vi "UHR-Fleezers Control (fpga) - 10.0.vi"() -> ()   [LabVIEW 2009]
doc: "UHR-Fleezers Instrument Control Code (fpga)"
uses:
  <vilib>/Platform/TimedLoop/XDataNode/XDataNode.xnode
  <vilib>/Platform/TimedLoop/XDataNode/loadlvalarms.vi
  <vilib>/Platform/TimedLoop/XDataNode/timing_clust.ctl
  <vilib>/Platform/TimedLoop/XDataNode/nitl_modes.ctl
  <vilib>/Platform/TimedLoop/XDataNode/wakeup.ctl
  <vilib>/eio/EIONode/EIONode.xnode
  <vilib>/rvi/eio/nirviEIOImplementation/nirviEIOImplementation.xnode
  <vilib>/rvi/eio/common/nirviEmuTemplateMethod_noerrors.vi
  <vilib>/rvi/eio/common/nirviEmuClasses.ctl
  <vilib>/eio/EIOMethodNode/EIOMethodNode.xnode
  <vilib>/rvi/eio/nirviEIOMethodImplementation/nirviEIOMethodImplementation.xnode
  <vilib>/rvi/DataTransferAndStorage/Container/XNode/niFpgaContainer.xnode
  <vilib>/rvi/interface/RandomDataEmulation/niFpgaRandomDataHandleErrors.vi
  <vilib>/rvi/interface/RandomDataEmulation/nirviRandomDataFPGAFIFO.vi
  <vilib>/rvi/DataTransferAndStorage/Container/Common/niFpgaContainerMethod.ctl
  <vilib>/rvi/DataTransferAndStorage/Container/Common/niFpgaTransferTypeControl.ctl
  <vilib>/addons/control/pid/fpga.llb/XNode/niFpgaPID.xnode
  <vilib>/Platform/TimedLoop/XDataNode/XDNodeRunTimeDep.lvlib
panel:
  out "AI1 X Set 2":i16
  in  "Tab Control":T1(tab)
  in  "Trap Pos FB Monitor T1 or T2":bool
  in  "Trap Pos FB Negate Action":bool
  in  "Trap Pos. FB SP":i16
  in  "Trap Pos. FB Reset":bool
  in  "Trap Pos to FIFO":bool
  in  "AI Averages":u16=1 min=1 step=1
  in  "AI1 Sets to FIFO":T2={"Set 1"=TRUE, "Set 2"=TRUE, "Set 3"=FALSE}
  in  "N of AI1 Int Acq Sets":i16=2 min=1 max=3 step=1
  out "Number of AI channels":i16
  out "AI Late Counter":u32
  in  "ai count":u32=400
  out "AI late?":bool
  in  "+ phase":bool
  in  "Phase count adjustment":i16
  out "Relative phase":i16
  in  "DMA buffer timeout":i32
  in  "AI to FIFO":bool
  out "BD1 Frequency Out 1":u64
  out "BD1 Frequency Out 2":u64
  in  "Force feedback":bool
  out "AI1 X Set 1":i16
  in  "Trap Pos. FB Gains":T3={"proportional gain (Kc)"=0.0, "integral gain (Kc*Ts/Ti)"=10.0, "derivative gain (Kc*Td/Ts)"=0.0} {"proportional gain (Kc)" format="%.11g"; "integral gain (Kc*Ts/Ti)" format="%.11g"; "derivative gain (Kc*Td/Ts)" format="%.11g"}
  in  "Trap Pos. FB Range":T4={"output high"=32767.0, "output low"=-32768.0}
  in  "Trap Pos. FB Mult Factor":i64=8589934592
  in  "Trap Pos. FB Offset Factor":i64
  in  "Tab Control 2":T5(tab)
  in  "Swap F1 and F2":bool
  in  "Freq or Amp switch first":bool=TRUE
  in  "Cont. Scan":bool
  in  "Abort scan":bool
  in  "Cycles per step":u64
  in  "Scan BD":bool
  in  "Number of scans":u16
  in  "Scan steps":u64
  in  "Scan freq.  increment":i64
  out "Scanning":bool
  in  "Start scan":bool
  in  "OSK Bd 1":bool
  in  "Reset Bd 1":bool
  in  "RD":bool
  in  "PMODE":bool
  in  "OSK Bd 2":bool
  in  "Reset Bd 2":bool
  in  "Direct RF Box \nCommunication":bool
  in  "Data BD 2":u8 format="%08b"
  in  "Data BD 1":u8 format="%08b"
  in  "Address":u8 format="%02x"
  in  "Update Data":bool
  in  "FPGA Controls\n RF Box":bool
  in  "Number Interlace Cycles":u8=2 min=1 max=3
  in  "Interlace Off Parameters":u8=1 min=1 max=3
  in  "Interlace ON/OFF":bool
  out "DIO Relative phase":i16
  in  "Phase count adjustment (DIO)":i16
  in  "+ phase (DIO)":bool
  out "DIO Late Counter":u32
  out "DIO Late?":bool
  in  "DIO count 1 (ticks)":u32=400
  in  "DIO count 2 (ticks)":u32=400
  in  "DIO count 3 (ticks)":u32=400
  out "AI2 Y Sum Set 2":i16
  out "AI2 Y Sum Set 1":i16
  in  "FB Gains Set 1":T6={"proportional gain (Kc)"=10, "integral gain (Kc*Ts/Ti)"=5, "derivative gain (Kc*Td/Ts)"=0}
  in  "FB Setpoint Set 1":i16 min=0 step=1
  in  "FB Reset Set 1":bool
  in  "FB On/Off Set 1":bool
  in  "FB Reset Set 2":bool
  in  "FB On/Off Set 2":bool
  in  "FB Setpoint Set 2":i16 min=0 step=1
  in  "FB Gains Set 2":T6={"proportional gain (Kc)"=10, "integral gain (Kc*Ts/Ti)"=5, "derivative gain (Kc*Td/Ts)"=0}
  in  "FB output range 2":cluster{"output high":i16, "output low":i16}={"output high"=3000, "output low"=0}
  in  "FB output range 1":cluster{"output high":i16, "output low":i16}={"output high"=3000, "output low"=0}
  out "Scan I":u64
  in  "Amp switch delay":u16=5
  in  "Freq switch delay":u16
  in  "BD 2 Amplitude 1":u16
  in  "BD 1 Amplitude 1":u16
  in  "BD 2 Frequency 1":u64
  in  "BD 1 Frequency 1":u64
  in  "BD 2 Amplitude 2":u16
  in  "BD 1 Amplitude 2":u16
  in  "BD 2 Frequency 2":u64
  in  "BD 1 Frequency 2":u64
  in  "BD 2 Amplitude 3":u16
  in  "BD 1 Amplitude 3":u16
  in  "BD 2 Frequency 3":u64
  in  "BD 1 Frequency 3":u64
  out "Numeric":i32
  out "AO2 2":i16
  out "AO1 2":i16
  in  "1D or 2D Scan?":bool
  in  "Abort scan (MCL)":bool
  in  "MCL Scan Axis":bool
  in  "Cont. Scan (MCL)":bool
  out "Scan I (MCL)":u64
  in  "Number of scans (MCL)":u16
  out "Scanning MCL":bool
  in  "Scan steps (MCL)":u64
  in  "Cycles per step (MCL)":u64
  in  "Scan freq.  increment (MCL)":i16
  in  "Start scan (MCL)":bool
  in  "AO2":i16
  in  "AO1":i16
  out "MCL Late Counter":u32
  out "MCL Late?":bool
  in  "MCL count":u32=800
  out "MCL Relative Phase":i16
  in  "Phase count adjustment (MCL)":i16
  in  "+ phase (MCL)":bool
  in  "APD2 Trigger on Edge?":bool=TRUE
  in  "APD1 Trigger on Edge?":bool=TRUE
  in  "APD Gate Operating Mode":u8 max=2 step=1
  in  "Invert APD Gate":bool
  in  "APD Gate OFF Count":u32=100
  in  "APD Gate ON Count":u32=300
  out "APD 1 Gate Late Counter":u32
  out "APD 1 Gate Late?":bool
  out "APD 1 Gate Relative Phase":i16
  in  "Phase count adjustment (APD 1 Gate)":i16
  in  "+ phase (APD 1 Gate)":bool
  out "APD 2 Counts 0":u32
  out "APD 2 Counts 1":u32
  out "APD 1 Counts 0":u32
  out "APD 1 Counts 1":u32
  out "APD out state":bool
  in  "APD 2 AO offset":i16
  in  "APD 1 AO offset":i16
  in  "APD 2 AO scale factor":i16=1
  in  "APD 1 AO scale factor":i16=1
  in  "APD to FIFO":bool
  in  "APD Acq Rate Count":u32=20000000
  out "APD Acq Late Counter":u32
  out "APD Acq Late?":bool
  out "APD Acq Relative Phase":i16
  in  "Phase Count Adjustment (APD Acq)":i16
  in  "+ phase (APD Acq)":bool
  in  "Phase count adjustment (APD 2 Gate)":i16
  out "APD 2 Gate Late Counter":u32
  out "APD 2 Gate Late?":bool
  out "APD 2 Gate Relative Phase":i16
  in  "+ phase (APD 2 Gate)":bool
  in  "Green Filter Flipper":bool
  out "Green FB Signals":T7
  in  "Green FB Count":u32=1200
  out "Green Late Counter":u32
  out "Green FB Late?":bool
  out "Green FB Relative Phase":i16
  in  "Phase count adjustment (Green FB)":i16=10
  in  "+ phase (Green FB)":bool
  out "Green FB Sum":i16
  in  "Green int current ON count adj":u32=150
  in  "Current Out":u16=30000
  in  "Green FB On/Off":bool
  in  "Green FB Setpoint":i16=250 min=0 step=1
  in  "Green FB Gains":T6={"proportional gain (Kc)"=10, "integral gain (Kc*Ts/Ti)"=5, "derivative gain (Kc*Td/Ts)"=0}
  in  "Green FB Reset":bool
  in  "Operating Mode 2":u8=2 max=2 step=1
  in  "Invert GI 2":bool
  in  "Green interlace OFF count 2":u32=900
  in  "Green interlace ON count 2":u32=300
  out "GI Late Counter 2":u32
  out "GI Late? 2":bool
  out "GI Relative phase 2":i16
  in  "Phase count adjustment (GI) 2":i16=20
  in  "+ phase (GI) 2":bool
  in  "Green interlace OFF count":u32=100
  out "GI Relative phase":i16
  in  "Phase count adjustment (GI)":i16
  in  "+ phase (GI)":bool
  out "GI Late?":bool
  in  "Green interlace ON count":u32=300
  out "GI Late Counter":u32
  in  "Invert GI":bool
  in  "Operating Mode":u8 max=2 step=1
  in  "Connector0/DIO9":bool
  in  "Connector1/DIO32":bool
  in  "Connector1/DIO33":bool
  in  "Connector1/DIO34":bool
  in  "Chassis2/Mod4/AO1":u16
  in  "Extra DO Counts":u32=40000
  # "Only one of these can be on\nat a time:"
  # "Raster Scan AOD"
  # "1 (X)"
  # "2 (Y)"
  # "IR Intensity Feedback (RF BD 1)"
  # "AO1 (Y)"
  # "2D"
  # "1D"
  # "AO2 (X)"
  # "APD AO for aligning"
  # "Detection Loop"
  # "Green fluorescent laser digital gate interlacing loop"
  # "0 Forced ON\n1 Forced OFF\n2 Interlacing"
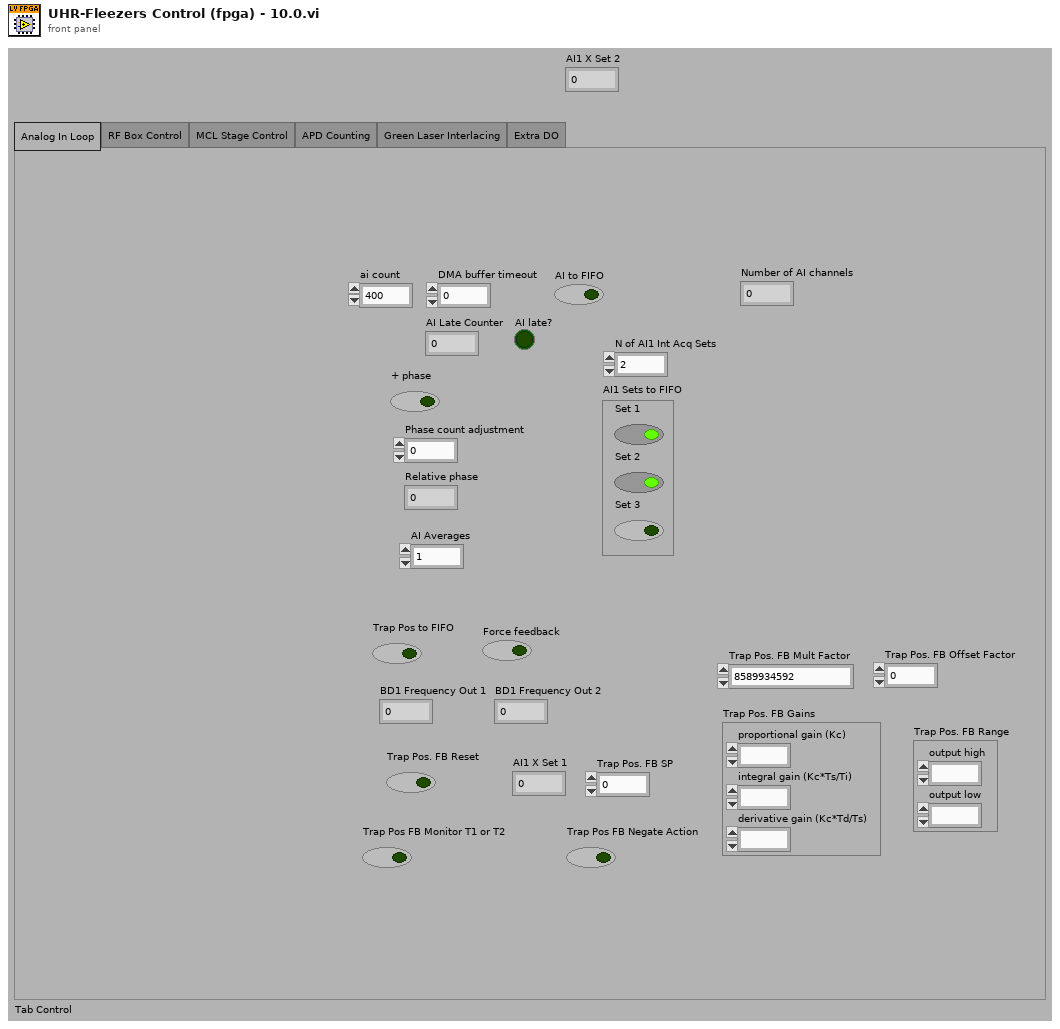
[diagram p1: front panel]
types:
  T1 = enum32{"Analog In Loop", "RF Box Control", "MCL Stage Control", "APD Counting", "Green Laser Interlacing", "Extra DO"}
  T2 = cluster{"Set 1":bool, "Set 2":bool, "Set 3":bool}
  T3 = cluster{"proportional gain (Kc)":fxp<+/-,16,8>, "integral gain (Kc*Ts/Ti)":fxp<+/-,16,8>, "derivative gain (Kc*Td/Ts)":fxp<+/-,16,8>}
  T4 = cluster{"output high":fxp<+/-,16,16>, "output low":fxp<+/-,16,16>}
  T5 = enum32{"Controls", "Interlacing Frequency and Amplitude Values"}
  T6 = cluster{"proportional gain (Kc)":i16, "integral gain (Kc*Ts/Ti)":i16, "derivative gain (Kc*Td/Ts)":i16}
  T7 = cluster{"Green FB Ch 0":i16, "Green FB Ch 1":i16, "Green FB Ch 2":i16}
  T8 = typedef "nirviEmuClasses.ctl" = enum16{"IO Read", "IO Write", "Method", "Property Read", "Property Write"}
  T9 = typedef "XDNodeRunTimeDep.lvlib/timing_clust.ctl" = cluster{"Expected End [f-1]":u64, "Actual End [f-1]":u64, "Finished Late? [f-1]":bool, "Expected End [i-1]":u64, "Actual End [i-1]":u64, "Finished Late? [i-1]":bool, "Expected Start [i]":u64, "Actual Start [i]":u64, "Expected Start [f]":u64, "Actual Start [f]":u64, "Source Name":string, "Structure Name":string, "Period":i64, "Deadline":i64, "Offset":i64, "Start":i64, "Priority":i32, "Timeout":i32, "Mode":T10, "Wakeup Reason":T11, "Error":errorcluster, "Source Type":string, "Secondary Source Type":string, "Global End Time":u64, "Global Start Time":u64, "Frame Duration":u64, "Iteration Duration":u64, "Assigned CPU":i32, "I/O Scan Engine Mode":u32}
  T10 = typedef "XDNodeRunTimeDep.lvlib/nitl_modes.ctl" = enum32{"No Change", "Process missed periods, maintain original phase", "Discard missed periods, maintain original phase", "Process missed periods, ignore original phase", "Discard missed periods, ignore original phase"}
  T11 = typedef "XDNodeRunTimeDep.lvlib/wakeup.ctl" = enum32{"Normal", "Aborted", "Asynchronous wakeup", "Timing source error", "Timed loop error", "Timeout"}
  T12 = typedef "niFpgaContainerMethod.ctl" = enum16{"Write", "Read", "Clear", "Get Number of Elements to Write", "Get Number of Elements to Read", "Enable", "Disable", "Flush and Disable", "Get Stream State"}
  T13 = typedef "niFpgaTransferTypeControl.ctl" = enum16{"Target-Scoped", "Host to Target - DMA", "Target to Host - DMA", "Peer to Peer Reader", "Peer to Peer Writer", "Bidirectional"}
  T14 = cluster{"Chassis2/Mod1/AI0":i16, "Chassis2/Mod1/AI1":i16, "Chassis2/Mod1/AI2":i16}
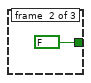
[diagram p2: hidden frame]
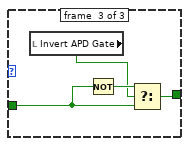
[diagram p3: hidden frame]
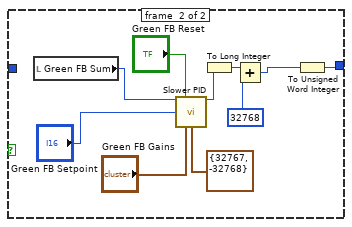
[diagram p4: hidden frame]
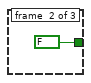
[diagram p5: hidden frame]
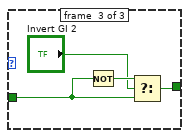
[diagram p6: hidden frame]
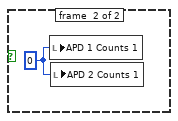
[diagram p7: hidden frame]
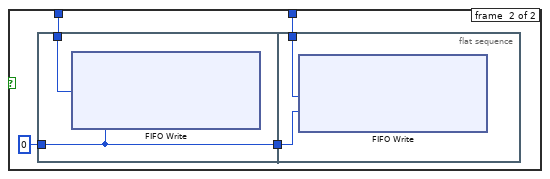
[diagram p8: hidden frame]
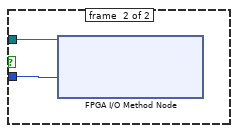
[diagram p9: hidden frame]
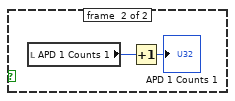
[diagram p10: hidden frame]
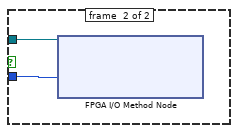
[diagram p11: hidden frame]
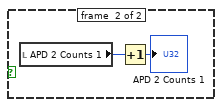
[diagram p12: hidden frame]
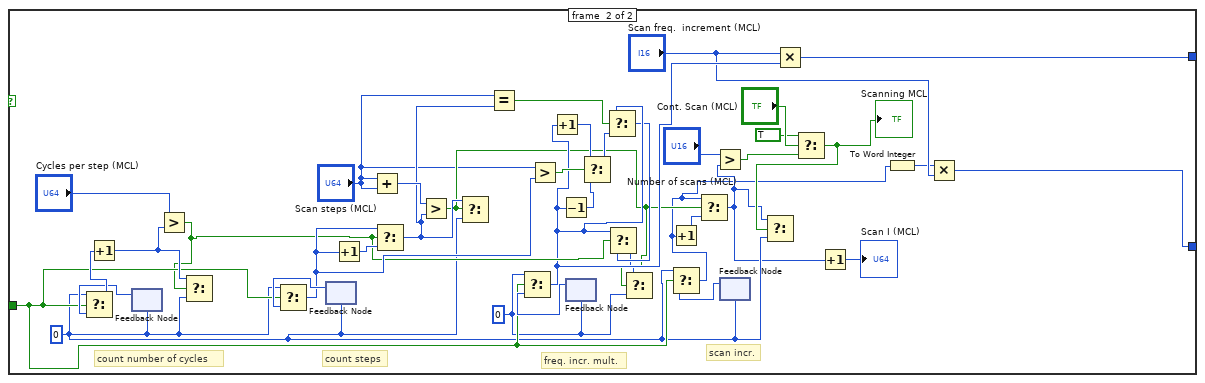
[diagram p13: hidden frame]
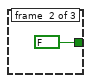
[diagram p14: hidden frame]
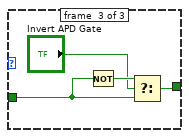
[diagram p15: hidden frame]
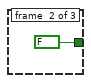
[diagram p16: hidden frame]
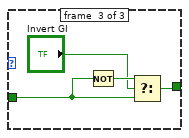
[diagram p17: hidden frame]
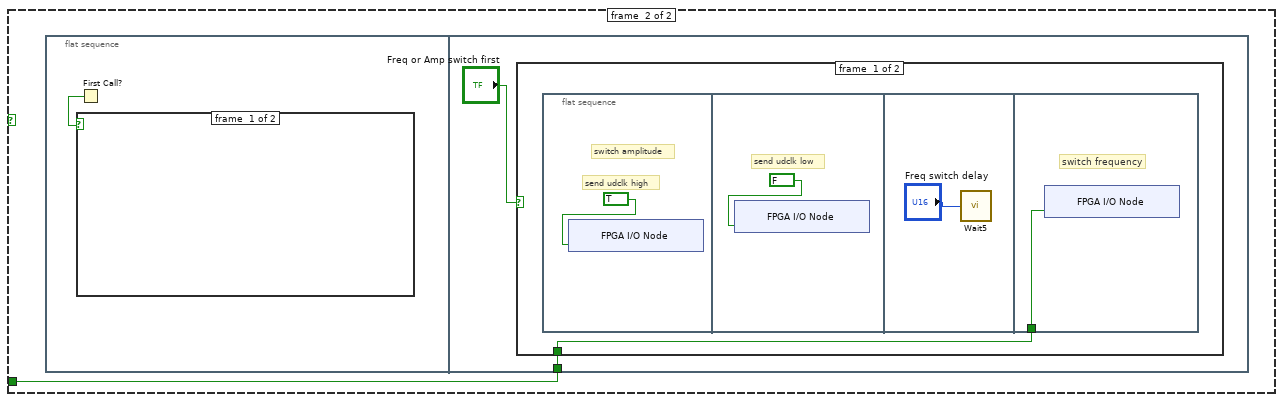
[diagram p18: hidden frame]
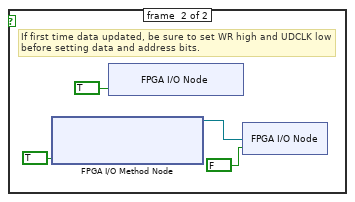
[diagram p19: hidden frame]
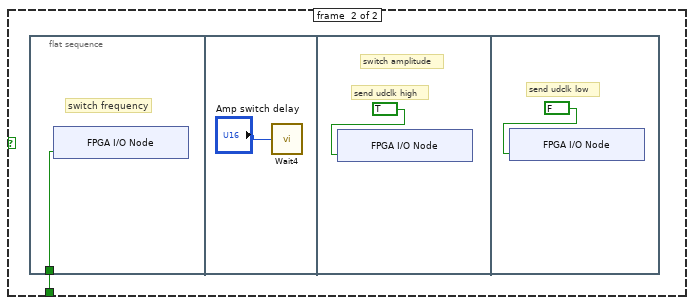
[diagram p20: hidden frame]
diagram:
  w2 = FALSE
  # "timing array current index"
  # "timing array"
  # "timing counter (phase adjusted here)"
  # "late counter"
  n1 = flat-sequence "FPGA initialization to do before running any of the loops" {
    tunnel: [u32 0 ("DIO count 3 (ticks)")] -> w1
    tunnel: [w10] -> _
    frame #0 {
      # "This is a kludge to let host programs know how many channels of data are in the DMA stream.  Set by hand."
      # "Start up expansion chassis early\nto avoid delays later"
      # "This pin controls udclk on the RF boards.\nWhen initially configuring the boards, this pin needs to be\nconfigured as a high impedance input.  Later it will be switched\nto an output."
      # "Initial setting of DIO data and \naddress to low (before reset).  \nThis needs to happen before the other\ncontrol method loops execute."
      n2 = xnode "FPGA I/O Node"("Chassis2/Mod4/AO0"=u16 0) -> ("Chassis2/Mod1/AI0"=w10:i16)  [unwired: 2 in, 2 out]
      n3 = xnode "FPGA I/O Method Node"("Enable"=FALSE) -> ()  [unwired: 1 in, 1 out]
      n4 = xnode "FPGA I/O Node"("Connector1/DIO0"=FALSE, "Connector1/DIO1"=FALSE, "Connector1/DIO2"=FALSE, "Connector1/DIO3"=FALSE, "Connector1/DIO4"=FALSE, "Connector1/DIO5"=FALSE, "Connector1/DIO6"=FALSE, "Connector1/DIO7"=FALSE, "Connector1/DIO8"=FALSE, "Connector1/DIO9"=FALSE, "Connector1/DIO10"=FALSE, "Connector1/DIO11"=FALSE, "Connector1/DIO12"=FALSE, "Connector1/DIO13"=FALSE, "Connector1/DIO15"=FALSE, "Connector1/DIO20"=FALSE, "Connector1/DIO21"=FALSE, "Connector1/DIO22"=FALSE, "Connector1/DIO23"=FALSE, "Connector1/DIO24"=FALSE, "Connector1/DIO25"=FALSE, "Connector1/DIO26"=FALSE, "Connector1/DIO27"=FALSE, "Connector1/DIO14"=FALSE) -> ()  [unwired: 24 in, 24 out]
      "Number of AI channels" <- i16 12 ("Number of AI channels")
    }
  }
  n5 = local read "AO1"() -> (w6:i16)
  n6 = local read "AO2"() -> (w5:i16)
  n7 = node-c288() -> (w4:T9)  [unwired: 1 in]
  n8 = while "APD 1 Counter" {
    tunnel: w1 -> [_]
    stop <- FALSE stop-if-true
    n9 = flat-sequence {
      frame #0 {
        n10 = case shown="False" "APD1 Trigger on Edge?" {
          tunnel: refnum<k21> "Connector0/DIO0" ("APD 1 DO") -> [w398 w423]
          tunnel: -1 ("Timeout") -> [w397 w422]
          frame #0 {
            n11 = xnode "FPGA I/O Method Node"("FPGA I/O In"=w398, "Timeout"=w397) -> ()  [unwired: 2 out]
          }
          frame #1 {
            n12 = xnode "FPGA I/O Method Node"("FPGA I/O In"=w423, "Timeout"=w422) -> ()  [unwired: 2 out]
          }
        }
      }
      frame #1 {
        n13 = local read "APD out state"() -> (w447:bool)
        n14 = case shown="False" w447 {
          frame #0 {
            n15 = local read "APD 1 Counts 0"() -> (w449:u32)
            n16 = Increment(x=w449) -> (x+1=→"APD 1 Counts 0":u32)
          }
          frame #1 {
            n17 = local read "APD 1 Counts 1"() -> (w451:u32)
            n18 = Increment(x=w451) -> (x+1=→"APD 1 Counts 1":u32)
          }
        }
      }
    }
  }
  n19 = while "APD 2 Counter" {
    tunnel: w1 -> [_]
    stop <- FALSE stop-if-true
    n20 = flat-sequence {
      frame #0 {
        n21 = case shown="False" "APD2 Trigger on Edge?" {
          tunnel: refnum<k21> "Connector0/DIO1" ("APD 2 DO") -> [w457 w482]
          tunnel: -1 ("Timeout") -> [w456 w481]
          frame #0 {
            n22 = xnode "FPGA I/O Method Node"("FPGA I/O In"=w457, "Timeout"=w456) -> ()  [unwired: 2 out]
          }
          frame #1 {
            n23 = xnode "FPGA I/O Method Node"("FPGA I/O In"=w482, "Timeout"=w481) -> ()  [unwired: 2 out]
          }
        }
      }
      frame #1 {
        n24 = local read "APD out state"() -> (w506:bool)
        n25 = case shown="False" w506 {
          frame #0 {
            n26 = local read "APD 2 Counts 0"() -> (w508:u32)
            n27 = Increment(x=w508) -> (x+1=→"APD 2 Counts 0":u32)
          }
          frame #1 {
            n28 = local read "APD 2 Counts 1"() -> (w510:u32)
            n29 = Increment(x=w510) -> (x+1=→"APD 2 Counts 1":u32)
          }
        }
      }
    }
  }
  n30 = while "APD 2 Gating" {
    shift-right: [w514] -> _
    shift-left: w1 -> [w519]
    shift-right: [w513] -> _
    shift-left: w2 -> [w511]
    stop <- FALSE stop-if-true
    n31 = flat-sequence {
      tunnel: w519 -> [w522]
      tunnel: [w523] -> w517
      tunnel: [w522] -> w515
      tunnel: [w521] -> w512
      tunnel: w511 -> [w521]
      tunnel: [w526] -> w518
      tunnel: w517 -> [w526]
      tunnel: [w525] -> w516
      tunnel: w515 -> [w525]
      tunnel: w512 -> [w524]
      tunnel: [w580] -> w514
      tunnel: w518 -> [w598]
      tunnel: w516 -> [w596]
      tunnel: [w585] -> w513
      frame #0 {
        n32 = call "Loop Timer8"("Count(Ticks)"=w522) -> ("Tick Count(Ticks)"=w523:u32)
      }
      frame #1 {
        # "(need 4 channels/APD)"
        n33 = xnode "FPGA I/O Node"("Connector0/DIO8"=w524, "Connector0/DIO9"=w524, "Connector0/DIO10"=w524, "Connector0/DIO11"=w524) -> ()  [unwired: 4 in, 4 out]
      }
      frame #2 {
        n34 = local read "APD Gate ON Count"() -> (w573:u32)
        n35 = local read "APD Gate OFF Count"() -> (w572:u32)
        n36 = feedback #1(TRUE) -> (w587:bool)
        n37 = feedback #2(w598) -> (w574:u32)
        n38 = Not(x=w587) -> (.not. x?=w584:bool)
        n39 = Subtract(x=w598, y=w574) -> (x-y=w597:u32)
        n40 = Select(t=w573, s=w584, f=w572) -> (s? t:f=w589:u32)
        n41 = Subtract(x=w597, y=w596) -> (x-y=w590:u32)
        n42 = Subtract(x=w589, y=w590) -> (x-y=w579:u32)
        n43 = Greater?(x=w590, y=u32 0) -> (0:w592:bool)
        "APD 2 Gate Late?" <- w592
        n44 = Boolean To (0,1)(Boolean="+ phase (APD 2 Gate)") -> (0, 1=w577:i16)
        n45 = Multiply(x=w577, y="Phase count adjustment (APD 2 Gate)") -> (x*y=w575:i16)
        n46 = feedback #3(u32 0) -> (w594:u32)
        n47 = Increment(x=w594) -> (x+1=w593:u32)
        n48 = Select(t=w593, s=w592, f=w594) -> (s? t:f=w591:u32)
        "APD 2 Gate Late Counter" <- w591
        n49 = Add(x=w579, y=w575) -> (x+y=w580:u32)
        n50 = feedback #4(i16 0) -> (w582:i16)
        n51 = Subtract(x=w582, y=w575) -> (x-y=w581:i16)
        "APD 2 Gate Relative Phase" <- w581
        n52 = local read "APD Gate Operating Mode"() -> (w571:u8)
        n53 = case shown="2" w571 {
          tunnel: [TRUE FALSE w604] -> w585
          tunnel: w587 -> [_ _ w602]
          frame #0 {
          }
          frame #1 {
          }
          frame #2 {
            n54 = local read "Invert APD Gate"() -> (w601:bool)
            n55 = Not(x=w602) -> (.not. x?=w603:bool)
            n56 = Select(t=w603, s=w601, f=w602) -> (s? t:f=w604:bool)
          }
        }
      }
    }
  }
  n57 = while "DAQ AI set 1" {
    shift-right: [w605] -> _
    shift-left: w1 -> [w610]
    stop <- FALSE stop-if-true
    n58 = flat-sequence {
      tunnel: w610 -> [w620]
      tunnel: [w621] -> w608
      tunnel: [w620] -> w607
      tunnel: [w631] -> w618
      tunnel: [w630] -> w617
      tunnel: [w629] -> w616
      tunnel: [w628] -> w615
      tunnel: [w627] -> w614
      tunnel: [w626] -> w613
      tunnel: [w625] -> w612
      tunnel: [w624] -> w611
      tunnel: [w623] -> w609
      tunnel: w608 -> [w623]
      tunnel: w607 -> [w622]
      tunnel: [w622] -> w606
      tunnel: [w813] -> w605
      tunnel: w618 -> [w849]
      tunnel: w617 -> [w805]
      tunnel: w616 -> [w833]
      tunnel: w615 -> [w848]
      tunnel: w614 -> [w837]
      tunnel: w613 -> [w836]
      tunnel: w612 -> [w835]
      tunnel: w611 -> [w834]
      tunnel: w609 -> [w830]
      tunnel: w606 -> [w827]
      frame #0 {
        n59 = call "Loop Timer3"("Count(Ticks)"=w620) -> ("Tick Count(Ticks)"=w621:u32)
      }
      frame #1 {
        n60 = xnode "FPGA I/O Node"("Connector1/DIO31"=TRUE ("Connector1/DIO33")) -> ("Connector0/AI0"=w631:i16, "Connector0/AI1"=w630:i16, "Connector0/AI2"=w629:i16, "Connector0/AI3"=w628:i16, "Connector0/AI4"=w627:i16, "Connector0/AI5"=w626:i16, "Connector0/AI6"=w625:i16, "Connector0/AI7"=w624:i16)  [unwired: 9 in, 9 out]
      }
      frame #2 {
        w808 = FALSE ("AI to FIFO")
        # "Adjust phase after data acquired if button pressed"
        n61 = feedback #5(i16 1) -> (w841:i16)
        n62 = Increment(x=w841) -> (x+1=w847:i16)
        n63 = Greater?(x=w847, y="N of AI1 Int Acq Sets") -> (0:w844:bool)
        n64 = Select(t=i16 1, s=w844, f=w847) -> (s? t:f=w846:i16)
        n65 = feedback #6(w808) -> (w806:bool)
        n66 = feedback #7(w808) -> (w832:bool)
        n67 = case shown="2" w841 {
          tunnel: w833 -> [w857 w892 _]
          tunnel: "AI1 Sets to FIFO" -> [w858 w893 w924]
          tunnel: [w855 w890 w923] -> w838
          tunnel: ["AI to FIFO" w889 w922] -> w831
          tunnel: w832 -> [_ w889 w922]
          tunnel: "DMA buffer timeout" -> [w856 w891 _]
          tunnel: ["Trap Pos to FIFO" w887 w921] -> w807
          tunnel: w806 -> [_ w887 w921]
          tunnel: w805 -> [w851 w886 _]
          frame #0 {
            n68 = Unbundle By Name(w858) -> ("Set 1"=w855:bool)
            n69 = Compound Arithmetic op=AND("Trap Pos to FIFO", w855, "AI to FIFO") -> (w853:bool)
            n70 = case shown="True" w853 {
              tunnel: w856 -> [_ w860]
              frame #0 {
              }
              frame #1 {
                n71 = local read "BD1 Frequency Out 1"() -> (w859:u64)
                n72 = xnode ("FIFO Method Node")("Element"=w859, "Timeout"=w860) -> ()  [unwired: 1 in, 2 out]
              }
            }
            "AI2 Y Sum Set 1" <- w857
            "AI1 X Set 1" <- w851
          }
          frame #1 {
            n73 = Unbundle By Name(w893) -> ("Set 2"=w890:bool)
            n74 = Compound Arithmetic op=AND(w887, w890, w889) -> (w888:bool)
            n75 = case shown="True" w888 {
              tunnel: w891 -> [_ w895]
              frame #0 {
              }
              frame #1 {
                n76 = local read "BD1 Frequency Out 2"() -> (w894:u64)
                n77 = xnode ("FIFO Method Node")("Element"=w894, "Timeout"=w895) -> ()  [unwired: 1 in, 2 out]
              }
            }
            "AI2 Y Sum Set 2" <- w892
            "AI1 X Set 2" <- w886
          }
          frame #2 {
            n78 = Unbundle By Name(w924) -> ("Set 3"=w923:bool)
          }
        }
        n79 = And(x=w838, y=w831) -> (x .and. y?=w840:bool)
        n80 = case shown="True" w840 {
          tunnel: w849 -> [_ w929]
          tunnel: w805 -> [_ w930]
          tunnel: w833 -> [_ w931]
          tunnel: w848 -> [_ w932]
          tunnel: w837 -> [_ w936]
          tunnel: w836 -> [_ w935]
          tunnel: w835 -> [_ w934]
          tunnel: w834 -> [_ w933]
          tunnel: "DMA buffer timeout" -> [_ w925]
          frame #0 {
          }
          frame #1 {
            n81 = Greater?(x="AI Averages", y=u16 1) -> (0:w927:bool)
            n82 = case shown="True" w927 {
              tunnel: w936 -> [w947 w1004]
              tunnel: w935 -> [w946 w1003]
              tunnel: w934 -> [w945 w1002]
              tunnel: w933 -> [w944 w1001]
              tunnel: w932 -> [w943 w1000]
              tunnel: w931 -> [w948 w999]
              tunnel: w930 -> [w949 w998]
              tunnel: w929 -> [w950 w997]
              tunnel: "AI Averages" -> [_ w984]
              tunnel: w925 -> [w938 w981]
              frame #0 {
                n83 = Join Numbers(hi=w950, lo=w949) -> ((hi.lo)=w942:u32)
                n84 = Join Numbers(hi=w948, lo=w943) -> ((hi.lo)=w941:u32)
                n85 = Join Numbers(hi=w947, lo=w946) -> ((hi.lo)=w940:u32)
                n86 = Join Numbers(hi=w945, lo=w944) -> ((hi.lo)=w939:u32)
                n87 = Build Array(w942, w941, w940, w939) -> (w937:u32[])
                n88 = for {
                  tunnel: w937 -> [w952] mode=indexing
                  tunnel: w938 -> [w953]
                  n89 = To Unsigned Long Integer(number=w952) -> (unsigned 32bit integer=w951:u32)
                  n90 = xnode ("FIFO Write")("Element"=w951, "Timeout"=w953) -> ()  [unwired: 1 in, 2 out]
                }
              }
              frame #1 {
                w988 = u16 0
                n91 = To Long Integer(number=w997) -> (32bit integer=w990:i32)
                n92 = To Long Integer(number=w998) -> (32bit integer=w1007:i32)
                n93 = To Long Integer(number=w999) -> (32bit integer=w1006:i32)
                n94 = To Long Integer(number=w1000) -> (32bit integer=w1005:i32)
                n95 = To Long Integer(number=w1004) -> (32bit integer=w996:i32)
                n96 = To Long Integer(number=w1003) -> (32bit integer=w995:i32)
                n97 = To Long Integer(number=w1002) -> (32bit integer=w994:i32)
                n98 = To Long Integer(number=w1001) -> (32bit integer=w993:i32)
                n99 = Build Array(w990, w1007, w1006, w1005, w996, w995, w994, w993) -> (w979:i32[])
                n100 = feedback #8(w979) -> (w992:i32[])
                n101 = Add(x=w979, y=w992) -> (x+y=w991:i32[])
                n102 = feedback #9(w988) -> (w986:u16)
                n103 = Increment(x=w986) -> (x+1=w983:u16)
                n104 = Equal?(x=w983, y=u16 1) -> (x = y?=w982:bool)
                n105 = Select(t=w979, s=w982, f=w991) -> (s? t:f=w980:i32[])
                n106 = Greater Or Equal?(x=w983, y=w984) -> (x >= y?=w985:bool)
                n107 = Select(t=w988, s=w985, f=w983) -> (s? t:f=w987:u16)
                n108 = case shown="True" w985 {
                  tunnel: w980 -> [_ w1009]
                  tunnel: w981 -> [_ w1008]
                  frame #0 {
                  }
                  frame #1 {
                    n109 = for {
                      tunnel: w1009 -> [w1011] mode=indexing
                      tunnel: w1008 -> [w1012]
                      n110 = To Unsigned Long Integer(number=w1011) -> (unsigned 32bit integer=w1010:u32)
                      n111 = xnode ("FIFO Write")("Element"=w1010, "Timeout"=w1012) -> ()  [unwired: 1 in, 2 out]
                    }
                  }
                }
              }
            }
          }
        }
        n112 = feedback #10(w830) -> (w829:u32)
        n113 = Subtract(x=w830, y=w829) -> (x-y=w828:u32)
        n114 = Subtract(x=w828, y=w827) -> (x-y=w824:u32)
        n115 = Subtract(x="ai count", y=w824) -> (x-y=w814:u32)
        n116 = Greater?(x=w824, y=u32 0) -> (0:w822:bool)
        "AI late?" <- w822
        n117 = xnode "I/O Node"("Connector1/DIO31"=FALSE ("Connector1/DIO34")) -> ()  [unwired: 1 in, 1 out]
        n118 = Boolean To (0,1)(Boolean="+ phase") -> (0, 1=w816:i16)
        n119 = feedback #11(u32 0) -> (w820:u32)
        n120 = Increment(x=w820) -> (x+1=w819:u32)
        n121 = Select(t=w819, s=w822, f=w820) -> (s? t:f=w821:u32)
        "AI Late Counter" <- w821
        n122 = Multiply(x=w816, y="Phase count adjustment") -> (x*y=w810:i16)
        n123 = feedback #12(i16 0) -> (w812:i16)
        n124 = Add(x=w814, y=w810) -> (x+y=w813:u32)
        n125 = Subtract(x=w812, y=w810) -> (x-y=w811:i16)
        "Relative phase" <- w811
      }
    }
  }
  n126 = while "RF box board DIO control: parallel communication" {
    shift-right: [w1057] -> _
    shift-left: w1 -> [w1056]
    shift-right: [w1055] -> _
    shift-left: FALSE ("Swap F1 and F2") -> [w1054]
    stop <- FALSE stop-if-true
    n127 = flat-sequence {
      tunnel: w1054 -> [w1061]
      tunnel: w1056 -> [w1059]
      tunnel: [w1061] -> w1053
      tunnel: [w1060] -> w1052
      tunnel: [w1059] -> w1051
      tunnel: [w1067] -> w1057
      tunnel: [w1066] -> w1055
      tunnel: w1053 -> [w1065]
      tunnel: w1052 -> [w1063]
      tunnel: w1051 -> [w1062]
      frame #0 {
        n128 = call "Loop Timer"("Count(Ticks)"=w1059) -> ("Tick Count(Ticks)"=w1060:u32)
      }
      frame #1 {
        n129 = flat-sequence {
          tunnel: ["FPGA Controls\n RF Box"] -> w1064
          tunnel: w1065 -> [w1068]
          tunnel: [w1217] -> w1067
          tunnel: [w1237] -> w1066
          tunnel: w1064 -> [w1236]
          tunnel: w1063 -> [w1230]
          tunnel: w1062 -> [w1227]
          frame #0 {
            n130 = case shown="True" "FPGA Controls\n RF Box" {
              tunnel: w1068 -> [_ w1070]
              frame #0 {
              }
              frame #1 {
                n131 = flat-sequence {
                  tunnel: w1070 -> [w1115]
                  frame #0 {
                    n132 = First Call?() -> (First Call?: T/F=w1071:bool)
                    n133 = case shown="True" w1071 {
                      frame #0 {
                      }
                      frame #1 {
                        # "If first time data updated, be sure to set WR high and UDCLK low\nbefore setting data and address bits."
                        n134 = xnode "FPGA I/O Method Node"("Enable"=TRUE) -> ("FPGA I/O Out"=w1073:refnum<k21>)  [unwired: 1 in]
                        n135 = xnode "FPGA I/O Node"("Connector1/DIO15"=TRUE) -> ()  [unwired: 1 in, 1 out]
                        n136 = xnode "FPGA I/O Node"("I/O Item"=FALSE ("Connector1/DIO30"), "FPGA I/O In"=w1073) -> ()  [unwired: 1 out]
                      }
                    }
                  }
                  frame #1 {
                    n137 = case shown="True" "Freq or Amp switch first" {
                      tunnel: w1115 -> [w1117 w1161]
                      frame #0 {
                        n138 = flat-sequence {
                          tunnel: w1117 -> [w1147]
                          frame #0 {
                            # "switch amplitude"
                            # "send udclk high"
                            n139 = xnode "FPGA I/O Node"("Connector1/DIO30"=TRUE ("Connector1/DIO15")) -> ()  [unwired: 1 in, 1 out]
                          }
                          frame #1 {
                            # "send udclk low"
                            n140 = xnode "FPGA I/O Node"("Connector1/DIO30"=FALSE ("Connector1/DIO15")) -> ()  [unwired: 1 in, 1 out]
                          }
                          frame #2 {
                            n141 = call "Wait5"("Count(Ticks)"="Freq switch delay") -> ()  [unwired: 1 out]
                          }
                          frame #3 {
                            # "switch frequency"
                            n142 = xnode "FPGA I/O Node"("Connector1/DIO36"=w1147) -> ()  [unwired: 1 in, 1 out]
                          }
                        }
                      }
                      frame #1 {
                        n143 = flat-sequence {
                          tunnel: w1161 -> [w1162]
                          frame #0 {
                            # "switch frequency"
                            n144 = xnode "FPGA I/O Node"("Connector1/DIO36"=w1162) -> ()  [unwired: 1 in, 1 out]
                          }
                          frame #1 {
                            n145 = call "Wait4"("Count(Ticks)"="Amp switch delay") -> ()  [unwired: 1 out]
                          }
                          frame #2 {
                            # "switch amplitude"
                            # "send udclk high"
                            n146 = xnode "FPGA I/O Node"("Connector1/DIO30"=TRUE ("Connector1/DIO15")) -> ()  [unwired: 1 in, 1 out]
                          }
                          frame #3 {
                            # "send udclk low"
                            n147 = xnode "FPGA I/O Node"("Connector1/DIO30"=FALSE ("Connector1/DIO15")) -> ()  [unwired: 1 in, 1 out]
                          }
                        }
                      }
                    }
                  }
                }
              }
            }
          }
          frame #1 {
            # "This is the prior cycle's on time"
            # "increment timing\nindex, reset to 0 if \nend of matrix"
            # "Reset to begginning (1) when number of cycles reached."
            # "timing index"
            # "build byte stacks for writing data\n(must correspond to addresses array constant)"
            # "Timing housekeeping"
            # "Adjust phase if late\n(maintains constant phase relationship between cycles)"
            n148 = feedback #13(u8 0 ("t")) -> (w1233:u8)
            n149 = Increment(x=w1233) -> (x+1=w1277:u8)
            n150 = Increment(x="Number Interlace Cycles") -> (x+1=w1272:u8)
            n151 = Equal?(x=w1277, y=w1272) -> (x = y?=w1279:bool)
            n152 = Select(t=u8 1, s=w1279, f=w1277) -> (s? t:f=w1232:u8)
            n153 = Increment(x=w1232) -> (x+1=w1274:u8)
            n154 = Equal?(x=w1274, y=w1272) -> (x = y?=w1275:bool)
            n155 = Select(t=u8 1, s=w1275, f=w1274) -> (s? t:f=w1271:u8)
            n156 = Select(t=w1271, s="Interlace ON/OFF", f="Interlace Off Parameters") -> (s? t:f=w1255:u8)
            n157 = case shown="1, Default" w1255 {
              tunnel: [w1354 "BD 1 Frequency 2" "BD 1 Frequency 3"] -> w1267
              tunnel: [w1353 "BD 2 Frequency 2" "BD 2 Frequency 3"] -> w1256
              tunnel: ["BD 2 Amplitude 1" "BD 2 Amplitude 2" "BD 2 Amplitude 3"] -> w1205
              tunnel: [w1342 w1466 "BD 1 Amplitude 3"] -> w1208
              frame #0 {
                w1349 = u64 0 ("f")
                # "Trap 1"
                n158 = local read "Scanning"() -> (w1355:bool)
                n159 = Or(x=w1355, y="Start scan") -> (x .or. y?=w1347:bool)
                n160 = Not(x="Abort scan") -> (.not. x?=w1345:bool)
                n161 = And(x=w1345, y=w1347) -> (x .and. y?=w1344:bool)
                n162 = case "For raster scanning" shown="False" w1344 {
                  tunnel: [u64 0 w1454] -> w1350
                  tunnel: "Start scan" -> [_ w1439]
                  frame #0 {
                    n163 = local write "Scanning"(FALSE ("scanning")) -> ()
                  }
                  frame #1 {
                    w1423 = i64 0
                    w1422 = u64 0
                    # "scan incr."
                    # "freq. incr. mult."
                    # "count steps"
                    # "count number of cycles"
                    n164 = feedback #14(w1422) -> (w1451:u64)
                    n165 = Select(t=w1422, s=w1439, f=w1451) -> (s? t:f=w1453:u64)
                    n166 = Increment(x=w1453) -> (x+1=w1450:u64)
                    n167 = Greater?(x="Cycles per step", y=w1450) -> (0:w1432:bool)
                    n168 = Select(t=w1450, s=w1432, f=w1422) -> (s? t:f=w1449:u64)
                    n169 = feedback #15(w1422) -> (w1448:u64)
                    n170 = Select(t=w1422, s=w1439, f=w1448) -> (s? t:f=w1443:u64)
                    n171 = Increment(x=w1443) -> (x+1=w1447:u64)
                    n172 = Add(x="Scan steps", y="Scan steps") -> (x+y=w1446:u64)
                    n173 = Select(t=w1443, s=w1432, f=w1447) -> (s? t:f=w1427:u64)
                    n174 = Greater?(x=w1446, y=w1427) -> (0:w1426:bool)
                    n175 = Select(t=w1427, s=w1426, f=w1422) -> (s? t:f=w1444:u64)
                    n176 = Equal?(x="Scan steps", y=w1427) -> (x = y?=w1431:bool)
                    n177 = Greater?(x="Scan steps", y=w1443) -> (0:w1442:bool)
                    n178 = feedback #16(w1423) -> (w1445:i64)
                    n179 = Select(t=w1423, s=w1439, f=w1445) -> (s? t:f=w1429:i64)
                    n180 = Increment(x=w1429) -> (x+1=w1441:i64)
                    n181 = Decrement(x=w1429) -> (x-1=w1440:i64)
                    n182 = Select(t=w1441, s=w1442, f=w1440) -> (s? t:f=w1430:i64)
                    n183 = Select(t=w1429, s=w1431, f=w1430) -> (s? t:f=w1428:i64)
                    n184 = Select(t=w1429, s=w1432, f=w1428) -> (s? t:f=w1424:i64)
                    n185 = Select(t=w1424, s=w1426, f=w1423) -> (s? t:f=w1425:i64)
                    n186 = feedback #17(w1422) -> (w1438:u64)
                    n187 = Select(t=w1422, s=w1439, f=w1438) -> (s? t:f=w1434:u64)
                    n188 = Increment(x=w1434) -> (x+1=w1435:u64)
                    n189 = Select(t=w1434, s=w1426, f=w1435) -> (s? t:f=w1433:u64)
                    n190 = Greater?(x="Number of scans", y=w1433) -> (0:w1419:bool)
                    n191 = Multiply(x="Scan freq.  increment", y=w1429) -> (x*y=w1454:i64)
                    n192 = Select(t=TRUE, s="Cont. Scan", f=w1419) -> (s? t:f=w1418:bool)
                    "Scanning" <- w1418
                    n193 = Select(t=w1433, s=w1418, f=w1422) -> (s? t:f=w1436:u64)
                    n194 = Increment(x=w1433) -> (x+1=→"Scan I":u64)
                  }
                }
                n195 = case "For position feedback" shown="True" "Force feedback" {
                  tunnel: [i64 0 w1368] -> w1339
                  frame #0 {
                  }
                  frame #1 {
                    # "2^33 (fixed point is like I16)\nexpands scale of output\nto full range of frequency spec\n(2^48)"
                    n196 = case shown="False" "Trap Pos FB Monitor T1 or T2" {
                      tunnel: [w1376 w1377] -> w1361
                      frame #0 {
                        n197 = local read "AI1 X Set 2"() -> (w1376:i16)
                      }
                      frame #1 {
                        n198 = local read "AI1 X Set 1"() -> (w1377:i16)
                      }
                    }
                    n199 = xnode ("PID")("process variable"=w1361, "reset?"="Trap Pos. FB Reset", "setpoint"="Trap Pos. FB SP", "PID gains"="Trap Pos. FB Gains", "output range"="Trap Pos. FB Range") -> ("output"=w1365:fxp<+/-,16,16>)
                    n200 = Negate(x=w1365) -> (-x=w1364:fxp<+/-,17,17>)
                    n201 = Select(t=w1364, s="Trap Pos FB Negate Action", f=w1365) -> (s? t:f=w1366:fxp<+/-,17,17>)
                    n202 = To Quad Integer(1:w1366) -> (0:w1371:i64)
                    n203 = Multiply(x=w1371, y="Trap Pos. FB Mult Factor") -> (x*y=w1369:i64)
                    n204 = Add(x=w1369, y="Trap Pos. FB Offset Factor") -> (x+y=w1368:i64)
                  }
                }
                n205 = case "For intensity feedback" shown="True" "FB On/Off Set 1" {
                  tunnel: "BD 1 Amplitude 1" -> [w1456 _]
                  tunnel: [w1456 w1457] -> w1342
                  frame #0 {
                  }
                  frame #1 {
                    n206 = local read "AI2 Y Sum Set 1"() -> (w1459:i16)
                    n207 = call "Slower PID.vi"("process variable"=w1459, "reset?"="FB Reset Set 1", "setpoint"="FB Setpoint Set 1", "PID gains (x 2^8)"="FB Gains Set 1", "output range"="FB output range 1") -> ("output"=w1462:i16)  [unwired: 10 out]
                    n208 = To Unsigned Word Integer(number=w1462) -> (unsigned 16bit integer=w1457:u16)
                  }
                }
                n209 = Select(t=w1349, s="Scan BD", f=w1350) -> (s? t:f=w1348:u64)
                n210 = Select(t=w1350, s="Scan BD", f=w1349) -> (s? t:f=w1351:u64)
                n211 = Add(x=w1348, y="BD 2 Frequency 1") -> (x+y=w1353:u64)
                n212 = Compound Arithmetic op=ADD("BD 1 Frequency 1", w1339, w1351) -> (w1354:u64)
                "BD1 Frequency Out 1" <- w1354
              }
              frame #1 {
                # "Trap 2"
                n213 = case shown="True" "FB On/Off Set 2" {
                  tunnel: [w1470 w1471] -> w1466
                  tunnel: "BD 1 Amplitude 2" -> [w1470 _]
                  frame #0 {
                  }
                  frame #1 {
                    n214 = local read "AI2 Y Sum Set 2"() -> (w1476:i16)
                    n215 = call "Slower PID.vi"("process variable"=w1476, "reset?"="FB Reset Set 2", "setpoint"="FB Setpoint Set 2", "PID gains (x 2^8)"="FB Gains Set 2", "output range"="FB output range 2") -> ("output"=w1473:i16)  [unwired: 10 out]
                    n216 = To Unsigned Word Integer(number=w1473) -> (unsigned 16bit integer=w1471:u16)
                  }
                }
                "BD1 Frequency Out 2" <- "BD 1 Frequency 2"
              }
              frame #2 {
                # "Fluorescence period"
              }
            }
            n217 = feedback #18(w1230) -> (w1229:u32)
            n218 = Subtract(x=w1230, y=w1229) -> (x-y=w1228:u32)
            n219 = Select(t=w1232, s="Interlace ON/OFF", f="Interlace Off Parameters") -> (s? t:f=w1270:u8)
            n220 = Subtract "The error"(x=w1228, y=w1227) -> (x-y=w1225:u32)
            n221 = case shown="3" w1270 {
              tunnel: ["DIO count 1 (ticks)" "DIO count 2 (ticks)" "DIO count 3 (ticks)"] -> w1226
              frame #0 {
              }
              frame #1 {
              }
              frame #2 {
              }
            }
            n222 = Greater?(x=w1225, y=u32 0) -> (0:w1220:bool)
            "DIO Late?" <- w1220
            n223 = feedback #19(u32 0) -> (w1222:u32)
            n224 = Increment(x=w1222) -> (x+1=w1221:u32)
            n225 = Select(t=w1221, s=w1220, f=w1222) -> (s? t:f=w1223:u32)
            "DIO Late Counter" <- w1223
            n226 = Subtract(x=w1226, y=w1225) -> (x-y=w1218:u32)
            n227 = Boolean To (0,1)(Boolean="+ phase (DIO)") -> (0, 1=w1215:i16)
            n228 = Multiply(x=w1215, y="Phase count adjustment (DIO)") -> (x*y=w1211:i16)
            n229 = feedback #20(i16 0) -> (w1213:i16)
            n230 = Subtract(x=w1213, y=w1211) -> (x-y=w1212:i16)
            "DIO Relative phase" <- w1212
            n231 = Split Number(x=w1267) -> (hi(x)=w1266:u32, lo(x)=w1265:u32)
            n232 = Split Number(x=w1256) -> (hi(x)=w1261:u32, lo(x)=w1260:u32)
            n233 = Split Number(x=w1266) -> (lo(x)=w1264:u16)  [unwired: 1 out]
            n234 = Split Number(x=w1265) -> (hi(x)=w1263:u16, lo(x)=w1262:u16)
            n235 = Split Number(x=w1261) -> (lo(x)=w1259:u16)  [unwired: 1 out]
            n236 = Split Number(x=w1260) -> (hi(x)=w1258:u16, lo(x)=w1257:u16)
            n237 = Split Number(x=w1208) -> (hi(x)=w1210:u8, lo(x)=w1209:u8)
            n238 = Split Number(x=w1205) -> (hi(x)=w1207:u8, lo(x)=w1206:u8)
            n239 = Add(x=w1218, y=w1211) -> (x+y=w1217:u32)
            n240 = Split Number(x=w1264) -> (hi(x)=w1254:u8, lo(x)=w1253:u8)
            n241 = Split Number(x=w1263) -> (hi(x)=w1252:u8, lo(x)=w1251:u8)
            n242 = Split Number(x=w1259) -> (hi(x)=w1247:u8, lo(x)=w1246:u8)
            n243 = Split Number(x=w1262) -> (hi(x)=w1250:u8, lo(x)=w1249:u8)
            n244 = Split Number(x=w1258) -> (hi(x)=w1245:u8, lo(x)=w1244:u8)
            n245 = Split Number(x=w1257) -> (hi(x)=w1243:u8, lo(x)=w1242:u8)
            n246 = Build Array "BD 1 A Stack"(w1210, w1209) -> (w1239:u8[])
            n247 = Build Array "BD 2 A Stack"(w1207, w1206) -> (w1238:u8[])
            n248 = Build Array "BD 1 nu Stack"(w1254, w1253, w1252, w1251, w1250, w1249) -> (w1248:u8[])
            n249 = Build Array "BD 2 nu Stack"(w1247, w1246, w1245, w1244, w1243, w1242) -> (w1241:u8[])
            n250 = case shown="2" w1255 {
              tunnel: [w1331 w1334] -> w1237
              tunnel: [u8 10 u8 4] -> w1240
              tunnel: "Swap F1 and F2" -> [w1332 w1334]
              frame #0 {
                # "F2"
                n251 = Not(x=w1332) -> (.not. x?=w1331:bool)
              }
              frame #1 {
                # "low chooses F1"
                # "F1"
              }
            }
            n252 = case "If FPGA is controlling (toggling) RF synth" shown="True" w1236 {
              tunnel: w1248 -> [_ w1284]
              tunnel: w1241 -> [_ w1283]
              tunnel: w1240 -> [_ w1282]
              tunnel: w1239 -> [_ w1281]
              tunnel: w1238 -> [_ w1280]
              frame #0 {
              }
              frame #1 {
                # "Write next amp.\n(wait until beginning of next loop iteration to update)"
                n253 = flat-sequence "Update the next F1 and F2 frequency value (the actual frequency won't change until FSK is switched).\nThen load the next amplitude value into buffer, but don't update it until the next cycle." {
                  tunnel: w1284 -> [w1287]
                  tunnel: w1283 -> [w1286]
                  tunnel: w1282 -> [w1285]
                  tunnel: w1281 -> [w1324]
                  tunnel: w1280 -> [w1323]
                  frame #0 {
                    n254 = for {
                      tunnel: w1287 -> [w1293] mode=indexing
                      tunnel: w1286 -> [w1292] mode=indexing
                      tunnel: w1285 -> [w1290]
                      i -> [w1291]
                      # "Write next freq."
                      n255 = To Unsigned Byte Integer(number=w1291) -> (unsigned 8bit integer=w1288:u8)
                      n256 = Add(x=w1290, y=w1288) -> (x+y=w1289:u8)
                      n257 = call "write to RF synth bd.vi"("Address Byte"=w1289, "BD 2 Byte"=w1292, "BD 1 Byte"=w1293) -> ()
                    }
                  }
                  frame #1 {
                    # "send udclk high"
                    n258 = xnode "FPGA I/O Node"("Connector1/DIO30"=TRUE ("Connector1/DIO15")) -> ()  [unwired: 1 in, 1 out]
                  }
                  frame #2 {
                    n259 = xnode "FPGA I/O Node"("Connector1/DIO30"=FALSE ("Connector1/DIO15")) -> ()  [unwired: 1 in, 1 out]
                  }
                  frame #3 {
                    n260 = for {
                      tunnel: w1324 -> [w1330] mode=indexing
                      tunnel: w1323 -> [w1329] mode=indexing
                      tunnel: u8 33 -> [w1327]
                      i -> [w1328]
                      n261 = To Unsigned Byte Integer(number=w1328) -> (unsigned 8bit integer=w1325:u8)
                      n262 = Add(x=w1327, y=w1325) -> (x+y=w1326:u8)
                      n263 = call "write to RF synth bd.vi"("Address Byte"=w1326, "BD 2 Byte"=w1329, "BD 1 Byte"=w1330) -> ()
                    }
                  }
                }
              }
            }
          }
        }
      }
    }
  }
  n264 = while "MCL stage control" {
    shift-right: [w1497] -> _
    shift-left: w1 -> [w1500]
    shift-right: [w1490] -> _
    shift-left: w6 -> [w1487]
    shift-right: [w1489] -> _
    shift-left: w5 -> [w1485]
    i -> [w1484]
    stop <- FALSE stop-if-true
    n265 = flat-sequence {
      tunnel: w1500 -> [w1504]
      tunnel: [w1505] -> w1496
      tunnel: [w1504] -> w1494
      tunnel: [w1503] -> w1488
      tunnel: w1487 -> [w1503]
      tunnel: [w1502] -> w1486
      tunnel: w1485 -> [w1502]
      tunnel: w1496 -> [w1509]
      tunnel: [w1509] -> w1495
      tunnel: w1494 -> [w1508]
      tunnel: [w1508] -> w1493
      tunnel: w1488 -> [w1507]
      tunnel: w1486 -> [w1506]
      tunnel: [w1507] -> w1483
      tunnel: [w1506] -> w1482
      tunnel: w1495 -> [w1543]
      tunnel: w1493 -> [w1542]
      tunnel: [w1543] -> w1499
      tunnel: [w1542] -> w1498
      tunnel: [w1541] -> w1492
      tunnel: [w1540] -> w1491
      tunnel: w1483 -> [w1535]
      tunnel: w1482 -> [w1534]
      tunnel: [w1607] -> w1497
      tunnel: w1499 -> [w1621]
      tunnel: w1498 -> [w1618]
      tunnel: w1492 -> [w1610]
      tunnel: w1491 -> [w1609]
      tunnel: [w1610] -> w1490
      tunnel: [w1609] -> w1489
      frame #0 {
        n266 = call "Loop Timer5"("Count(Ticks)"=w1504) -> ("Tick Count(Ticks)"=w1505:u32)
      }
      frame #1 {
        n267 = xnode "FPGA I/O Node"("Connector0/AO1"=w1507, "Connector0/AO2"=w1506) -> ()  [unwired: 2 in, 2 out]
      }
      frame #2 {
        n268 = local read "Scanning MCL"() -> (w1555:bool)
        n269 = Or(x=w1555, y="Start scan (MCL)") -> (x .or. y?=w1550:bool)
        n270 = Not(x="Abort scan (MCL)") -> (.not. x?=w1548:bool)
        n271 = And(x=w1548, y=w1550) -> (x .and. y?=w1547:bool)
        n272 = case "Raster scan" shown="True" w1547 {
          tunnel: [w1556 w1599] -> w1552
          tunnel: "Start scan (MCL)" -> [_ w1584]
          tunnel: [w1556 w1560] -> w1536
          frame #0 {
            w1556 = i16 0
            n273 = local write "Scanning MCL"(FALSE ("scanning")) -> ()
          }
          frame #1 {
            w1570 = i16 0
            w1569 = u64 0
            # "scan incr."
            # "freq. incr. mult."
            # "count steps"
            # "count number of cycles"
            n274 = feedback #21(w1569) -> (w1596:u64)
            n275 = Select(t=w1569, s=w1584, f=w1596) -> (s? t:f=w1598:u64)
            n276 = Increment(x=w1598) -> (x+1=w1595:u64)
            n277 = Greater?(x="Cycles per step (MCL)", y=w1595) -> (0:w1579:bool)
            n278 = Select(t=w1595, s=w1579, f=w1569) -> (s? t:f=w1594:u64)
            n279 = feedback #22(w1569) -> (w1593:u64)
            n280 = Select(t=w1569, s=w1584, f=w1593) -> (s? t:f=w1588:u64)
            n281 = Increment(x=w1588) -> (x+1=w1592:u64)
            n282 = Add(x="Scan steps (MCL)", y="Scan steps (MCL)") -> (x+y=w1591:u64)
            n283 = Select(t=w1588, s=w1579, f=w1592) -> (s? t:f=w1574:u64)
            n284 = Greater?(x=w1591, y=w1574) -> (0:w1573:bool)
            n285 = Select(t=w1574, s=w1573, f=w1569) -> (s? t:f=w1589:u64)
            n286 = Equal?(x="Scan steps (MCL)", y=w1574) -> (x = y?=w1578:bool)
            n287 = Greater?(x="Scan steps (MCL)", y=w1588) -> (0:w1587:bool)
            n288 = feedback #23(w1570) -> (w1590:i16)
            n289 = Select(t=w1570, s=w1584, f=w1590) -> (s? t:f=w1576:i16)
            n290 = Increment(x=w1576) -> (x+1=w1586:i16)
            n291 = Decrement(x=w1576) -> (x-1=w1585:i16)
            n292 = Select(t=w1586, s=w1587, f=w1585) -> (s? t:f=w1577:i16)
            n293 = Select(t=w1576, s=w1578, f=w1577) -> (s? t:f=w1575:i16)
            n294 = Select(t=w1576, s=w1579, f=w1575) -> (s? t:f=w1571:i16)
            n295 = Select(t=w1571, s=w1573, f=w1570) -> (s? t:f=w1572:i16)
            n296 = feedback #24(w1569) -> (w1583:u64)
            n297 = Select(t=w1569, s=w1584, f=w1583) -> (s? t:f=w1558:u64)
            n298 = Increment(x=w1558) -> (x+1=w1580:u64)
            n299 = Select(t=w1558, s=w1573, f=w1580) -> (s? t:f=w1559:u64)
            n300 = Greater?(x="Number of scans (MCL)", y=w1559) -> (0:w1566:bool)
            n301 = Multiply(x="Scan freq.  increment (MCL)", y=w1576) -> (x*y=w1599:i16)
            n302 = Select(t=TRUE, s="Cont. Scan (MCL)", f=w1566) -> (s? t:f=w1565:bool)
            "Scanning MCL" <- w1565
            n303 = Select(t=w1559, s=w1565, f=w1569) -> (s? t:f=w1581:u64)
            n304 = Increment(x=w1559) -> (x+1=→"Scan I (MCL)":u64)
            n305 = To Word Integer(number=w1558) -> (16bit integer=w1561:i16)
            n306 = Multiply(x=w1561, y="Scan freq.  increment (MCL)") -> (x*y=w1560:i16)
          }
        }
        n307 = Select(t=w1536, s="1D or 2D Scan?", f=i16 0) -> (s? t:f=w1537:i16)
        n308 = Select(t=w1537, s="MCL Scan Axis", f=w1552) -> (s? t:f=w1551:i16)
        n309 = Select(t=w1552, s="MCL Scan Axis", f=w1537) -> (s? t:f=w1553:i16)
        n310 = Add(x=w1551, y="AO2") -> (x+y=w1540:i16)
        n311 = Add(x="AO1", y=w1553) -> (x+y=w1541:i16)
        "AO1 2" <- w1535
        "AO2 2" <- w1534
      }
      frame #3 {
        n312 = feedback #25(w1621) -> (w1620:u32)
        n313 = Boolean To (0,1)(Boolean="+ phase (MCL)") -> (0, 1=w1605:i16)
        n314 = Subtract(x=w1621, y=w1620) -> (x-y=w1619:u32)
        n315 = Multiply(x=w1605, y="Phase count adjustment (MCL)") -> (x*y=w1601:i16)
        n316 = Subtract(x=w1619, y=w1618) -> (x-y=w1616:u32)
        n317 = Subtract(x="MCL count", y=w1616) -> (x-y=w1603:u32)
        n318 = feedback #26(i16 0) -> (w1602:i16)
        n319 = Subtract(x=w1602, y=w1601) -> (x-y=w1600:i16)
        "MCL Relative Phase" <- w1600
        n320 = Greater?(x=w1616, y=u32 0) -> (0:w1615:bool)
        "MCL Late?" <- w1615
        n321 = Add(x=w1603, y=w1601) -> (x+y=w1607:u32)
        n322 = feedback #27(u32 0) -> (w1613:u32)
        n323 = Increment(x=w1613) -> (x+1=w1612:u32)
        n324 = Select(t=w1612, s=w1615, f=w1613) -> (s? t:f=w1614:u32)
        "MCL Late Counter" <- w1614
      }
    }
    "Numeric" <- w1484
  }
  n325 = while "APD 1 Gating" {
    shift-right: [w1626] -> _
    shift-left: w1 -> [w1631]
    shift-right: [w1625] -> _
    shift-left: w2 -> [w1623]
    stop <- FALSE stop-if-true
    n326 = flat-sequence {
      tunnel: w1631 -> [w1634]
      tunnel: [w1635] -> w1629
      tunnel: [w1634] -> w1627
      tunnel: [w1633] -> w1624
      tunnel: w1623 -> [w1633]
      tunnel: [w1638] -> w1630
      tunnel: w1629 -> [w1638]
      tunnel: [w1637] -> w1628
      tunnel: w1627 -> [w1637]
      tunnel: w1624 -> [w1636]
      tunnel: [w1688] -> w1626
      tunnel: w1630 -> [w1710]
      tunnel: w1628 -> [w1707]
      tunnel: [w1693] -> w1625
      frame #0 {
        n327 = call "Loop Timer7"("Count(Ticks)"=w1634) -> ("Tick Count(Ticks)"=w1635:u32)
      }
      frame #1 {
        # "(need 4 channels/APD)"
        n328 = xnode "FPGA I/O Node"("Connector0/DIO4"=w1636, "Connector0/DIO5"=w1636, "Connector0/DIO6"=w1636, "Connector0/DIO7"=w1636) -> ()  [unwired: 4 in, 4 out]
      }
      frame #2 {
        n329 = feedback #28(TRUE) -> (w1696:bool)
        n330 = feedback #29(w1710) -> (w1709:u32)
        n331 = Not(x=w1696) -> (.not. x?=w1692:bool)
        n332 = Subtract(x=w1710, y=w1709) -> (x-y=w1708:u32)
        n333 = Select(t="APD Gate ON Count", s=w1692, f="APD Gate OFF Count") -> (s? t:f=w1698:u32)
        n334 = Subtract(x=w1708, y=w1707) -> (x-y=w1699:u32)
        n335 = Subtract(x=w1698, y=w1699) -> (x-y=w1687:u32)
        n336 = Greater?(x=w1699, y=u32 0) -> (0:w1703:bool)
        "APD 1 Gate Late?" <- w1703
        n337 = Boolean To (0,1)(Boolean="+ phase (APD 1 Gate)") -> (0, 1=w1685:i16)
        n338 = Multiply(x=w1685, y="Phase count adjustment (APD 1 Gate)") -> (x*y=w1683:i16)
        n339 = feedback #30(u32 0) -> (w1705:u32)
        n340 = Increment(x=w1705) -> (x+1=w1704:u32)
        n341 = Select(t=w1704, s=w1703, f=w1705) -> (s? t:f=w1702:u32)
        "APD 1 Gate Late Counter" <- w1702
        n342 = Add(x=w1687, y=w1683) -> (x+y=w1688:u32)
        n343 = feedback #31(i16 0) -> (w1690:i16)
        n344 = Subtract(x=w1690, y=w1683) -> (x-y=w1689:i16)
        "APD 1 Gate Relative Phase" <- w1689
        n345 = case shown="2" "APD Gate Operating Mode" {
          tunnel: [TRUE FALSE w1716] -> w1693
          tunnel: w1696 -> [_ _ w1713]
          frame #0 {
          }
          frame #1 {
          }
          frame #2 {
            n346 = Not(x=w1713) -> (.not. x?=w1715:bool)
            n347 = Select(t=w1715, s="Invert APD Gate", f=w1713) -> (s? t:f=w1716:bool)
          }
        }
      }
    }
  }
  n348 = while "RF box board direct communication loop" {
    tunnel: w1 -> [_]
    stop <- FALSE stop-if-true
    n349 = case "Whether to use direct communication method (only use one method at a time)" shown="True" "Direct RF Box \nCommunication" {
      frame #0 {
      }
      frame #1 {
        n350 = case shown="True" "Update Data" {
          frame #0 {
          }
          frame #1 {
            n351 = flat-sequence {
              frame #0 {
                n352 = First Call?() -> (First Call?: T/F=w1720:bool)
                n353 = case shown="True" w1720 {
                  frame #0 {
                  }
                  frame #1 {
                    # "If first time data updated, be sure to set WR high\nbefore setting data and address bits."
                    n354 = flat-sequence {
                      frame #0 {
                        n355 = xnode "FPGA I/O Node"("Connector1/DIO15"=TRUE) -> ()  [unwired: 1 in, 1 out]
                      }
                      frame #1 {
                        n356 = call "Wait"("Count(Ticks)"=u8 40 ("DO Delay 3 (Ticks)")) -> ()  [unwired: 1 out]
                      }
                    }
                  }
                }
              }
              frame #1 {
                n357 = Number To Boolean Array(number="Address") -> (Boolean array=w1782:bool[])
                n358 = Number To Boolean Array(number="Data BD 1") -> (Boolean array=w1783:bool[])
                n359 = Number To Boolean Array(number="Data BD 2") -> (Boolean array=w1752:bool[])
                n360 = Index Array(array=w1783, index=7) -> (element=w1767:bool)
                n361 = Index Array(array=w1783, index=6) -> (element=w1766:bool)
                n362 = Index Array(array=w1783, index=5) -> (element=w1765:bool)
                n363 = Index Array(array=w1783, index=4) -> (element=w1764:bool)
                n364 = Index Array(array=w1783, index=3) -> (element=w1763:bool)
                n365 = Index Array(array=w1783, index=2) -> (element=w1762:bool)
                n366 = Index Array(array=w1783, index=1) -> (element=w1761:bool)
                n367 = Index Array(array=w1783, index=0) -> (element=w1760:bool)
                n368 = Index Array(array=w1782, index=5) -> (element=w1759:bool)
                n369 = Index Array(array=w1782, index=4) -> (element=w1758:bool)
                n370 = Index Array(array=w1782, index=3) -> (element=w1757:bool)
                n371 = Index Array(array=w1782, index=2) -> (element=w1756:bool)
                n372 = Index Array(array=w1782, index=1) -> (element=w1755:bool)
                n373 = Index Array(array=w1782, index=0) -> (element=w1754:bool)
                n374 = Index Array(array=w1752, index=7) -> (element=w1743:bool)
                n375 = Index Array(array=w1752, index=6) -> (element=w1742:bool)
                n376 = Index Array(array=w1752, index=5) -> (element=w1741:bool)
                n377 = Index Array(array=w1752, index=4) -> (element=w1740:bool)
                n378 = Index Array(array=w1752, index=3) -> (element=w1739:bool)
                n379 = Index Array(array=w1752, index=2) -> (element=w1738:bool)
                n380 = Index Array(array=w1752, index=1) -> (element=w1737:bool)
                n381 = Index Array(array=w1752, index=0) -> (element=w1736:bool)
                n382 = xnode "FPGA I/O Node"("Connector1/DIO0"=w1767, "Connector1/DIO1"=w1766, "Connector1/DIO2"=w1765, "Connector1/DIO3"=w1764, "Connector1/DIO4"=w1763, "Connector1/DIO5"=w1762, "Connector1/DIO6"=w1761, "Connector1/DIO7"=w1760, "Connector1/DIO8"=w1759, "Connector1/DIO9"=w1758, "Connector1/DIO10"=w1757, "Connector1/DIO11"=w1756, "Connector1/DIO12"=w1755, "Connector1/DIO13"=w1754, "Connector1/DIO20"=w1743, "Connector1/DIO21"=w1742, "Connector1/DIO22"=w1741, "Connector1/DIO23"=w1740, "Connector1/DIO24"=w1739, "Connector1/DIO25"=w1738, "Connector1/DIO26"=w1737, "Connector1/DIO27"=w1736) -> ()  [unwired: 22 in, 22 out]
              }
              frame #2 {
                # "wait and then apply write signal"
                n383 = call "Wait2"("Count(Ticks)"=u8 40 ("DO Delay 1 (Ticks)")) -> ()  [unwired: 1 out]
              }
              frame #3 {
                # "sending bit low writes data to board buffer"
                n384 = xnode "FPGA I/O Node"("Connector1/DIO15"=FALSE) -> ()  [unwired: 1 in, 1 out]
              }
              frame #4 {
                # "wait then return write signal"
                n385 = call "Wait3"("Count(Ticks)"=u8 40 ("DO Delay 2 (Ticks)")) -> ()  [unwired: 1 out]
              }
              frame #5 {
                # "sending bit high makes ready to\nwrite more data"
                n386 = xnode "FPGA I/O Node"("Connector1/DIO15"=TRUE) -> ()  [unwired: 1 in, 1 out]
              }
            }
          }
        }
      }
    }
  }
  n387 = while "Control APD data integration - stream to host" {
    shift-right: [w2104] -> _
    shift-left: w1 -> [w2109]
    stop <- FALSE stop-if-true
    n388 = flat-sequence {
      tunnel: w2109 -> [w2111]
      tunnel: [w2112] -> w2107
      tunnel: [w2111] -> w2105
      tunnel: [w2120] -> w2108
      tunnel: w2107 -> [w2120]
      tunnel: [w2119] -> w2106
      tunnel: w2105 -> [w2119]
      tunnel: [w2118] -> w2103
      tunnel: [w2117] -> w2102
      tunnel: [w2144] -> w2104
      tunnel: w2108 -> [w2169]
      tunnel: w2106 -> [w2166]
      tunnel: w2103 -> [w2137]
      tunnel: w2102 -> [w2136]
      frame #0 {
        n389 = call "Loop Timer6"("Count(Ticks)"=w2111) -> ("Tick Count(Ticks)"=w2112:u32)
      }
      frame #1 {
        n390 = flat-sequence {
          tunnel: [w2121] -> w2116
          tunnel: w2116 -> [w2124]
          tunnel: [w2126] -> w2115
          tunnel: [w2125] -> w2114
          tunnel: [w2124] -> w2113
          tunnel: [w2132] -> w2117
          tunnel: [w2133] -> w2118
          tunnel: w2115 -> [w2133]
          tunnel: w2114 -> [w2132]
          tunnel: w2113 -> [w2131]
          frame #0 {
            n391 = feedback #32(FALSE) -> (w2122:bool)
            "APD out state" <- w2122
            n392 = Not(x=w2122) -> (.not. x?=w2121:bool)
          }
          frame #1 {
            n393 = local read "APD 1 Counts 1"() -> (w2130:u32)
            n394 = local read "APD 1 Counts 0"() -> (w2129:u32)
            n395 = local read "APD 2 Counts 1"() -> (w2128:u32)
            n396 = local read "APD 2 Counts 0"() -> (w2127:u32)
            n397 = Select(t=w2130, s=w2124, f=w2129) -> (s? t:f=w2126:u32)
            n398 = Select(t=w2128, s=w2124, f=w2127) -> (s? t:f=w2125:u32)
          }
          frame #2 {
            n399 = case shown="False" w2131 {
              frame #0 {
                w2134 = u32 0 ("APD 1 Counts 0")
                n400 = local write "APD 1 Counts 0"(w2134) -> ()
                n401 = local write "APD 2 Counts 0"(w2134) -> ()
              }
              frame #1 {
                w2135 = u32 0 ("APD 1 Counts 1")
                n402 = local write "APD 1 Counts 1"(w2135) -> ()
                n403 = local write "APD 2 Counts 1"(w2135) -> ()
              }
            }
          }
        }
      }
      frame #2 {
        n404 = feedback #33(w2169) -> (w2168:u32)
        n405 = Subtract(x=w2169, y=w2168) -> (x-y=w2167:u32)
        n406 = Subtract(x=w2167, y=w2166) -> (x-y=w2160:u32)
        n407 = case shown="True" "APD to FIFO" {
          tunnel: w2137 -> [_ w2196]
          tunnel: w2136 -> [_ w2194]
          frame #0 {
          }
          frame #1 {
            n408 = flat-sequence {
              tunnel: 0 ("Timeout") -> [w2198]
              tunnel: w2196 -> [w2199]
              tunnel: [w2198] -> w2195
              tunnel: w2195 -> [w2226]
              tunnel: w2194 -> [w2225]
              frame #0 {
                n409 = xnode ("FIFO Write")("Element"=w2199, "Timeout"=w2198) -> ()  [unwired: 1 in, 2 out]
              }
              frame #1 {
                n410 = xnode ("FIFO Write")("Element"=w2225, "Timeout"=w2226) -> ()  [unwired: 1 in, 2 out]
              }
            }
          }
        }
        n411 = Subtract(x="APD Acq Rate Count", y=w2160) -> (x-y=w2145:u32)
        n412 = Greater?(x=w2160, y=u32 0) -> (0:w2162:bool)
        "APD Acq Late?" <- w2162
        n413 = feedback #34(u32 0) -> (w2164:u32)
        n414 = Increment(x=w2164) -> (x+1=w2163:u32)
        n415 = Select(t=w2163, s=w2162, f=w2164) -> (s? t:f=w2161:u32)
        "APD Acq Late Counter" <- w2161
        n416 = Boolean To (0,1)(Boolean="+ phase (APD Acq)") -> (0, 1=w2141:i16)
        n417 = Multiply(x=w2141, y="Phase Count Adjustment (APD Acq)") -> (x*y=w2138:i16)
        n418 = Add(x=w2145, y=w2138) -> (x+y=w2144:u32)
        n419 = feedback #35(i16 0) -> (w2143:i16)
        n420 = Subtract(x=w2143, y=w2138) -> (x-y=w2140:i16)
        "APD Acq Relative Phase" <- w2140
        n421 = To Word Integer(number=w2137) -> (16bit integer=w2153:i16)
        n422 = To Word Integer(number=w2136) -> (16bit integer=w2154:i16)
        n423 = Multiply(x="APD 1 AO scale factor", y=w2153) -> (x*y=w2152:i16)
        n424 = Multiply(x="APD 2 AO scale factor", y=w2154) -> (x*y=w2151:i16)
        n425 = Add(x="APD 1 AO offset", y=w2152) -> (x+y=w2150:i16)
        n426 = Add(x=w2151, y="APD 2 AO offset") -> (x+y=w2148:i16)
        n427 = xnode "FPGA I/O Node"("Connector0/AO6"=w2150, "Connector0/AO7"=w2148) -> ()  [unwired: 2 in, 2 out]
      }
    }
  }
  n428 = timed-loop "RF box board DIO control: control bits" {
    timing: w4 -> [_]
    timing-out: [_] -> w3
    tunnel: [w2252] -> _
    tunnel: w1 -> [w2252]
    stop <- FALSE stop-if-true
    n429 = xnode "FPGA I/O Node"("Connector1/DIO16"="RD", "Connector1/DIO17"="PMODE", "Connector1/DIO18"="OSK Bd 1", "Connector1/DIO19"="Reset Bd 1", "Connector1/DIO28"="OSK Bd 2", "Connector1/DIO29"="Reset Bd 2") -> ()  [unwired: 6 in, 6 out]
  }
  n430 = while "Green fluorescent laser interlacing (DO to IA 532 nm AOM ME amp)." {
    shift-right: [w2343] -> _
    shift-left: w1 -> [w2348]
    shift-right: [w2342] -> _
    shift-left: FALSE -> [w2340]
    stop <- FALSE stop-if-true
    n431 = flat-sequence {
      tunnel: w2348 -> [w2351]
      tunnel: [w2352] -> w2346
      tunnel: [w2351] -> w2344
      tunnel: [w2350] -> w2341
      tunnel: w2340 -> [w2350]
      tunnel: [w2355] -> w2347
      tunnel: w2346 -> [w2355]
      tunnel: [w2354] -> w2345
      tunnel: w2344 -> [w2354]
      tunnel: w2341 -> [w2353]
      tunnel: [w2395] -> w2343
      tunnel: w2347 -> [w2422]
      tunnel: w2345 -> [w2419]
      tunnel: [w2405] -> w2342
      frame #0 {
        n432 = call "Loop Timer4"("Count(Ticks)"=w2351) -> ("Tick Count(Ticks)"=w2352:u32)
      }
      frame #1 {
        n433 = xnode "FPGA I/O Node"("Connector1/DIO37"=w2353, "Connector1/DIO38"=w2353, "Connector1/DIO39"=w2353) -> ()  [unwired: 3 in, 3 out]
      }
      frame #2 {
        n434 = feedback #36(w2422) -> (w2421:u32)
        n435 = Subtract(x=w2422, y=w2421) -> (x-y=w2420:u32)
        n436 = Subtract(x=w2420, y=w2419) -> (x-y=w2411:u32)
        n437 = Greater?(x=w2411, y=u32 0) -> (0:w2415:bool)
        "GI Late?" <- w2415
        n438 = Boolean To (0,1)(Boolean="+ phase (GI)") -> (0, 1=w2400:i16)
        n439 = Multiply(x=w2400, y="Phase count adjustment (GI)") -> (x*y=w2397:i16)
        n440 = feedback #37(u32 0) -> (w2417:u32)
        n441 = Increment(x=w2417) -> (x+1=w2416:u32)
        n442 = Select(t=w2416, s=w2415, f=w2417) -> (s? t:f=w2414:u32)
        "GI Late Counter" <- w2414
        n443 = feedback #38(i16 0) -> (w2398:i16)
        n444 = Subtract(x=w2398, y=w2397) -> (x-y=w2396:i16)
        "GI Relative phase" <- w2396
        n445 = feedback #39(TRUE) -> (w2408:bool)
        n446 = case shown="2" "Operating Mode" {
          tunnel: [TRUE FALSE w2428] -> w2405
          tunnel: w2408 -> [_ _ w2425]
          frame #0 {
          }
          frame #1 {
          }
          frame #2 {
            n447 = Not(x=w2425) -> (.not. x?=w2427:bool)
            n448 = Select(t=w2427, s="Invert GI", f=w2425) -> (s? t:f=w2428:bool)
          }
        }
        n449 = Not(x=w2408) -> (.not. x?=w2404:bool)
        n450 = Select(t="Green interlace ON count", s=w2404, f="Green interlace OFF count") -> (s? t:f=w2410:u32)
        n451 = Subtract(x=w2410, y=w2411) -> (x-y=w2401:u32)
        n452 = Add(x=w2401, y=w2397) -> (x+y=w2395:u32)
      }
    }
  }
  n453 = while "Green fluorescent laser interlacing (Current to IA 532 nm AOM ME amp)." {
    shift-right: [w2434] -> _
    shift-left: w1 -> [w2437]
    shift-right: [w2431] -> _
    shift-left: w1 -> [w2429]
    stop <- FALSE stop-if-true
    n454 = flat-sequence {
      tunnel: w2437 -> [w2440]
      tunnel: [w2441] -> w2436
      tunnel: [w2440] -> w2435
      tunnel: [w2439] -> w2430
      tunnel: w2429 -> [w2439]
      tunnel: [w2444] -> w2433
      tunnel: w2436 -> [w2444]
      tunnel: [w2443] -> w2432
      tunnel: w2435 -> [w2443]
      tunnel: w2430 -> [w2442]
      tunnel: [w2457] -> w2434
      tunnel: [w2475] -> w2431
      tunnel: w2433 -> [w2494]
      tunnel: w2432 -> [w2491]
      frame #0 {
        n455 = call "Loop Timer10"("Count(Ticks)"=w2440) -> ("Tick Count(Ticks)"=w2441:u32)
      }
      frame #1 {
        n456 = xnode "FPGA I/O Node"("Chassis2/Mod4/AO0"=w2442) -> ()  [unwired: 1 in, 1 out]
      }
      frame #2 {
        n457 = Subtract(x="Green interlace OFF count 2", y="Green int current ON count adj") -> (x-y=w2467:u32)
        n458 = feedback #40(w2494) -> (w2493:u32)
        n459 = Add(x="Green int current ON count adj", y="Green interlace ON count 2") -> (x+y=w2468:u32)
        n460 = Subtract(x=w2494, y=w2493) -> (x-y=w2492:u32)
        n461 = Subtract(x=w2492, y=w2491) -> (x-y=w2483:u32)
        n462 = Greater?(x=w2483, y=u32 0) -> (0:w2487:bool)
        "GI Late? 2" <- w2487
        n463 = Boolean To (0,1)(Boolean="+ phase (GI) 2") -> (0, 1=w2463:i16)
        n464 = Multiply(x=w2463, y="Phase count adjustment (GI) 2") -> (x*y=w2459:i16)
        n465 = feedback #41(u32 0) -> (w2489:u32)
        n466 = Increment(x=w2489) -> (x+1=w2488:u32)
        n467 = Select(t=w2488, s=w2487, f=w2489) -> (s? t:f=w2486:u32)
        "GI Late Counter 2" <- w2486
        n468 = feedback #42(i16 0) -> (w2460:i16)
        n469 = Subtract(x=w2460, y=w2459) -> (x-y=w2458:i16)
        "GI Relative phase 2" <- w2458
        n470 = feedback #43(TRUE) -> (w2480:bool)
        n471 = case shown="2" "Operating Mode 2" {
          tunnel: [TRUE FALSE w2511] -> w2469
          tunnel: w2480 -> [_ _ w2508]
          frame #0 {
          }
          frame #1 {
          }
          frame #2 {
            n472 = Not(x=w2508) -> (.not. x?=w2510:bool)
            n473 = Select(t=w2510, s="Invert GI 2", f=w2508) -> (s? t:f=w2511:bool)
          }
        }
        n474 = And(x=w2469, y="Green FB On/Off") -> (x .and. y?=w2470:bool)
        n475 = case shown="True" w2470 {
          tunnel: "Current Out" -> [w2495 _]
          tunnel: [w2495 w2500] -> w2474
          frame #0 {
          }
          frame #1 {
            n476 = local read "Green FB Sum"() -> (w2496:i16)
            n477 = call "Slower PID.vi"("process variable"=w2496, "reset?"="Green FB Reset", "setpoint"="Green FB Setpoint", "PID gains (x 2^8)"="Green FB Gains", "output range"=cluster{"output high":i16, "output low":i16} {"output high"=32767, "output low"=-32768} ("Green FB output range")) -> ("output"=w2504:i16)  [unwired: 10 out]
            n478 = To Long Integer(number=w2504) -> (32bit integer=w2497:i32)
            n479 = Add(x=w2497, y=32768) -> (x+y=w2499:i32)
            n480 = To Unsigned Word Integer(number=w2499) -> (unsigned 16bit integer=w2500:u16)
          }
        }
        n481 = Not(x=w2480) -> (.not. x?=w2477:bool)
        n482 = Select(t=w2468, s=w2477, f=w2467) -> (s? t:f=w2482:u32)
        n483 = Subtract(x=w2482, y=w2483) -> (x-y=w2461:u32)
        n484 = Add(x=w2461, y=w2459) -> (x+y=w2457:u32)
        n485 = Boolean To (0,1)(Boolean=w2469) -> (0, 1=w2476:i16)
        n486 = To Unsigned Word Integer(number=w2476) -> (unsigned 16bit integer=w2473:u16)
        n487 = Multiply(x=w2473, y=w2474) -> (x*y=w2475:u16)
      }
    }
  }
  n488 = while "Green excitation laser feedback measurement" {
    shift-right: [w2512] -> _
    shift-left: w1 -> [w2517]
    stop <- FALSE stop-if-true
    n489 = flat-sequence {
      tunnel: w2517 -> [w2519]
      tunnel: [w2520] -> w2515
      tunnel: [w2519] -> w2513
      tunnel: [w2527] -> w2516
      tunnel: w2515 -> [w2527]
      tunnel: [w2526] -> w2514
      tunnel: w2513 -> [w2526]
      tunnel: [w2603] -> w2512
      tunnel: w2516 -> [w2621]
      tunnel: w2514 -> [w2618]
      frame #0 {
        n490 = call "Loop Timer9"("Count(Ticks)"=w2519) -> ("Tick Count(Ticks)"=w2520:u32)
      }
      frame #1 {
        n491 = xnode "FPGA I/O Node"("Connector1/DIO35"=TRUE) -> ("Chassis2/Mod1/AI0"=w2525:i16, "Chassis2/Mod1/AI1"=w2524:i16, "Chassis2/Mod1/AI2"=w2521:i16)  [unwired: 4 in, 4 out]
        "Green FB Sum" <- w2521
        n492 = Bundle("Chassis2/Mod1/AI0"=w2525, "Chassis2/Mod1/AI1"=w2524, "Chassis2/Mod1/AI2"=w2521) -> (→"Green FB Signals":T14)  [unwired: 1 out]
      }
      frame #2 {
        n493 = feedback #44(w2621) -> (w2620:u32)
        n494 = Subtract(x=w2621, y=w2620) -> (x-y=w2619:u32)
        n495 = xnode "FPGA I/O Node"("Connector1/DIO35"=FALSE) -> ()  [unwired: 1 in, 1 out]
        n496 = Subtract(x=w2619, y=w2618) -> (x-y=w2612:u32)
        n497 = Subtract(x="Green FB Count", y=w2612) -> (x-y=w2607:u32)
        n498 = Greater?(x=w2612, y=u32 0) -> (0:w2614:bool)
        "Green FB Late?" <- w2614
        n499 = Boolean To (0,1)(Boolean="+ phase (Green FB)") -> (0, 1=w2605:i16)
        n500 = Multiply(x=w2605, y="Phase count adjustment (Green FB)") -> (x*y=w2600:i16)
        n501 = feedback #45(u32 0) -> (w2616:u32)
        n502 = Increment(x=w2616) -> (x+1=w2615:u32)
        n503 = Select(t=w2615, s=w2614, f=w2616) -> (s? t:f=w2613:u32)
        "Green Late Counter" <- w2613
        n504 = Add(x=w2607, y=w2600) -> (x+y=w2603:u32)
        n505 = feedback #46(i16 0) -> (w2602:i16)
        n506 = Subtract(x=w2602, y=w2600) -> (x-y=w2601:i16)
        "Green FB Relative Phase" <- w2601
      }
    }
  }
  n507 = while "Control Additional IO (Green laser flip mount)" {
    stop <- FALSE stop-if-true
    n508 = xnode "FPGA I/O Node"("Connector0/DIO3"="Green Filter Flipper", "Connector0/DIO2"="Connector0/DIO9", "Connector1/DIO32"="Connector1/DIO32", "Connector1/DIO33"="Connector1/DIO33", "Connector1/DIO34"="Connector1/DIO34", "Chassis2/Mod4/AO1"="Chassis2/Mod4/AO1") -> ()  [unwired: 6 in, 6 out]
    n509 = call "Loop Timer2"("Count(Ticks)"="Extra DO Counts") -> ()  [unwired: 1 out]
  }
  n510 = node-c288(w3) -> ()
